vi "IV_RLJ_2015640305_P5.vi"(7 "OPERACIONES":T2(ring), 8 "Error In":errorcluster, 10 "OPERADORES":T1 {"y 2" scale=0.0..4.0; "Meter" scale=-360.0..360.0 scale format="%#_3g"; "y" scale=-150.0..150.0; "x" scale=-150.0..150.0}, 11 "IMAGEN 1":path) -> (0 "Error Out":errorcluster, 1 "HISTOGRAMA":dbl[][](graph), 2 "IMAGEN MODIFICADA":picture, 3 "IMAGEN ORIGINAL":picture)   [LabVIEW 2016]
doc: "subVI para la operacion sobre imagenes jpg, jpeg, o png que muestra el histograma RGB de la imagen modificada."
uses:
  <vilib>/picture/picture.llb/Draw True-Color Pixmap.vi
  <vilib>/imath/engines/lvmath2/RunTimeEngine/Managers/WorkSpace/UID Generator.vi
  <vilib>/imath/engines/lvmath2/RunTimeEngine/BuiltInFunctions/size/NIMS_[I32,I32]=size(GM).vi
  <instcachedir>/0/NIMS_[I32,I32]=size(GM)_B0A6EC1255BB4C8AB801FE6F734128D9.lvgen/NIMS_[I32,I32]=size(GM)_B0A6EC1255BB4C8AB801FE6F734128D9_005.vi
  <vilib>/imath/engines/lvmath2/RunTimeSupport/NIMS_Complex To Real.vi
  <instcachedir>/0/NIMS_Complex To Real_A9DD49CC305F495FA24B9F5762C73A31.lvgen/NIMS_Complex To Real_A9DD49CC305F495FA24B9F5762C73A31_001.vi
  <vilib>/imath/engines/lvmath2/RunTimeEngine/BuiltInFunctions/zeros/NIMS_M=zeros(I32,I32).vi
  <vilib>/imath/engines/lvmath2/RunTimeEngine/ErrorHandling/NIMS_Create Error From Enums.vi
  <vilib>/imath/engines/lvmath2/RunTimeEngine/RangeToken/NIMS_Range.vi
  <instcachedir>/0/NIMS_Range_A7C094595B484CA7AF10685B02D808ED.lvgen/NIMS_Range_A7C094595B484CA7AF10685B02D808ED_000.vi
  <vilib>/imath/engines/lvmath2/RunTimeSupport/NIMS_Error if Not Equal.vi
  <instcachedir>/0/NIMS_Error if Not Equal_43252A79AD05436189442EC0C5E5AB8A.lvgen/NIMS_Error if Not Equal_43252A79AD05436189442EC0C5E5AB8A_001.vi
  <vilib>/imath/engines/lvmath2/RunTimeEngine/IndexReplace/NIMS M(V,V)=M.vi
  <instcachedir>/0/NIMS M(V,V)=M_7C673E496ABD4677A4D7F51E7F4F45D1.lvgen/NIMS M(V,V)=M_7C673E496ABD4677A4D7F51E7F4F45D1_004.vi
  <vilib>/imath/engines/lvmath2/RunTimeEngine/BuiltInFunctions/size/NIMS_I32=size(GM,I32).vi
  <instcachedir>/0/NIMS_I32=size(GM,I32)_122058B1B3294FAEA5DC209B92B394E4.lvgen/NIMS_I32=size(GM,I32)_122058B1B3294FAEA5DC209B92B394E4_005.vi
  <vilib>/imathl/engines/lvmath/Functions/Error Handling/Create Error.vi
  <vilib>/imath/engines/lvmath2/RunTimeEngine/BuiltInFunctions/size/NIMS_I32Row=size(GM).vi
  <instcachedir>/0/NIMS_I32Row=size(GM)_10ACDCB9F1F84A7E9F42C91D87611FB5.lvgen/NIMS_I32Row=size(GM)_10ACDCB9F1F84A7E9F42C91D87611FB5_006.vi
  <vilib>/imath/engines/lvmath2/RunTimeEngine/BuiltInFunctions/zeros/NIMS_M=zeros(I32V).vi
  <vilib>/imath/engines/lvmath2/RunTimeEngine/RangeToken/NIMS_Range_R2 - Integer.vi
  <instcachedir>/0/NIMS_Range_R2 - Integer_89B873E74E6E489885E44F751DD9C6BF.lvgen/NIMS_Range_R2 - Integer_89B873E74E6E489885E44F751DD9C6BF_000.vi
  <vilib>/imath/engines/lvmath2/RunTimeEngine/CommandStatement/MC_CommandStatement_break.vi
  <vilib>/imath/engines/lvmath2/RunTimeEngine/BuiltInFunctions/round/NIMS_round(DBL-S).vi
  <instcachedir>/0/NIMS_Error if Not Equal_43252A79AD05436189442EC0C5E5AB8A.lvgen/NIMS_Error if Not Equal_43252A79AD05436189442EC0C5E5AB8A_000.vi
  <vilib>/imath/engines/lvmath2/RunTimeEngine/IndexRead/NIMS M(S,S).vi
  <instcachedir>/0/NIMS M(S,S)_AC51E74150A542F7991B9634C66F3096.lvgen/NIMS M(S,S)_AC51E74150A542F7991B9634C66F3096_002.vi
  <vilib>/imath/engines/lvmath2/RunTimeEngine/IndexReplace/NIMS M(S,S)=S.vi
  <instcachedir>/0/NIMS M(S,S)=S_98E40400474E4398B113AE20298B4F82.lvgen/NIMS M(S,S)=S_98E40400474E4398B113AE20298B4F82_003.vi
  <vilib>/imath/engines/lvmath2/RunTimeEngine/RunTimeType/NIMS_RunTimeType_From StrictType (excl LVString).vi
  <instcachedir>/0/NIMS_RunTimeType_From StrictType (excl LVString)_BBF44FB49F834B71AF7A14CCEDF8BECD.lvgen/NIMS_RunTimeType_From StrictType (excl LVString)_BBF44FB49F834B71AF7A14CCEDF8BECD_000.vi
  <vilib>/imath/engines/lvmath2/RunTimeEngine/LocalVariableDefStatement/MC_LocalVariableDefStatement_Display.vi
  <vilib>/imath/engines/lvmath2/RunTimeEngine/IndexRead/NIMS M(V,V).vi
  <instcachedir>/0/NIMS M(V,V)_DD7FAD36288F49D588C120E7830B6EC1.lvgen/NIMS M(V,V)_DD7FAD36288F49D588C120E7830B6EC1_005.vi
  <vilib>/imath/engines/lvmath2/RunTimeEngine/Managers/SymbolTable/Clear UID.vi
  <vilib>/imath/engines/lvmath2/RunTimeEngine/NodeEndStatement/NIMS_NodeEndStatement_Output.vi
  <instcachedir>/0/NIMS_NodeEndStatement_Output_53EC0D466D134D7ABD903AC30B43404B.lvgen/NIMS_NodeEndStatement_Output_53EC0D466D134D7ABD903AC30B43404B_010.vi
  <vilib>/imath/engines/lvmath2/RunTimeEngine/ErrorHandling/NIMS_Finalize Error.vi
  <vilib>/Analysis/Matrix/Numeric/Conversions/Array To Matrix - RA2.vi
  <vilib>/Analysis/Matrix/Numeric/Conversions/Matrix To Array - RM.vi
  <vilib>/imath/engines/lvmath2/RunTimeEngine/BuiltInFunctions/rotate90/NIMS_rotate90.vi
  <instcachedir>/0/NIMS_rotate90_7DC1660D109944E092D2EB6E3185A1B6.lvgen/NIMS_rotate90_7DC1660D109944E092D2EB6E3185A1B6_004.vi
  <vilib>/imath/engines/lvmath2/RunTimeEngine/IndexRead/NIMS M(R2,S).vi
  <instcachedir>/0/NIMS M(R2,S)_56813DCFDD5A484292D2195AF15D2BF5.lvgen/NIMS M(R2,S)_56813DCFDD5A484292D2195AF15D2BF5_000.vi
  <vilib>/imath/engines/lvmath2/RunTimeEngine/IndexReplace/NIMS M(R2,S)=V.vi
  <instcachedir>/0/NIMS M(R2,S)=V_4CAA475A15784754AE70E3CCB958AE2E.lvgen/NIMS M(R2,S)=V_4CAA475A15784754AE70E3CCB958AE2E_000.vi
  <instcachedir>/0/NIMS_NodeEndStatement_Output_53EC0D466D134D7ABD903AC30B43404B.lvgen/NIMS_NodeEndStatement_Output_53EC0D466D134D7ABD903AC30B43404B_002.vi
  <vilib>/Analysis/Matrix/NI_Matrix.lvlib
  <vilib>/imath/engines/lvmath2/RunTimeEngine/Managers/SymbolTable/NIMS_WorkSpace.lvlib
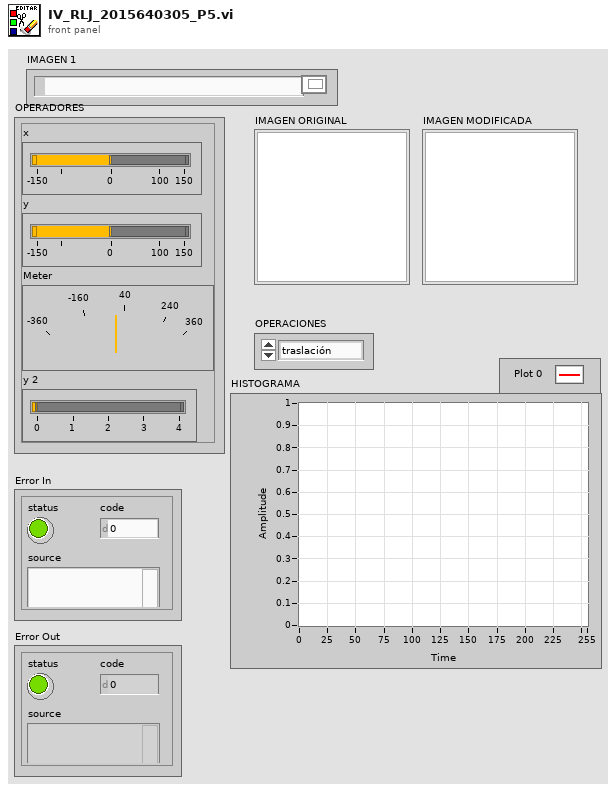
[diagram p1: front panel]
types:
  T1 = cluster{"x":dbl, "y":dbl, "Meter":dbl, "y 2":i64}
  T2 = enum16{"traslación", "Rotación", "Zoom", "GIROH", "GIROV", "Extracción", "Sustitución", "UNION"}
  T3 = typedef "imagedata.ctl" = cluster{"image type":i32, "image depth":i32, "image":u8[], "mask":u8[], "colors":u32[], "Rectangle":cluster{"left":i16, "top":i16, "right":i16, "bottom":i16}}
  T4 = typedef "NI_Matrix.lvlib/RealMatrix.ctl" = dbl[][]
  T5 = cluster{"left":i16, "top":i16, "right":i16, "bottom":i16}
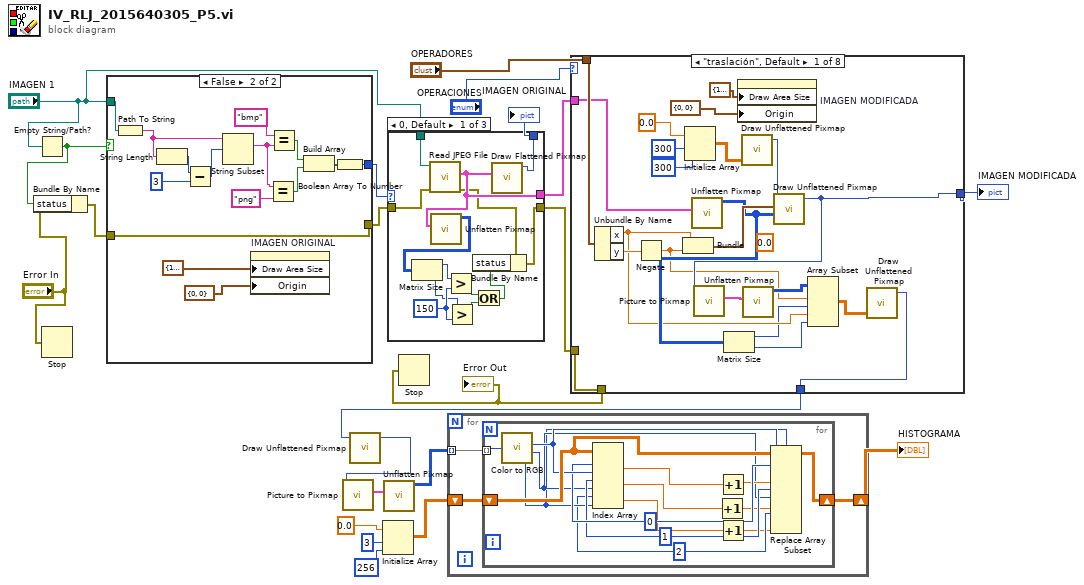
[diagram p0: block diagram]
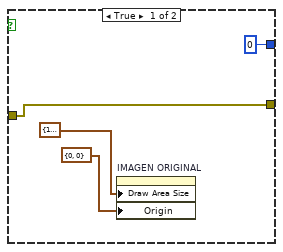
[diagram p2: hidden frame]
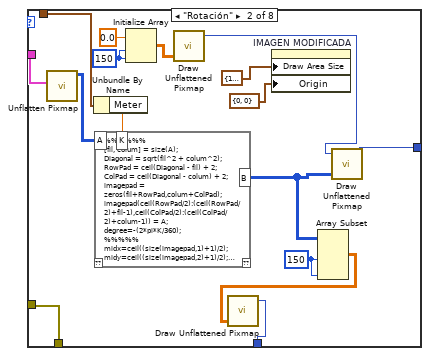
[diagram p3: hidden frame]
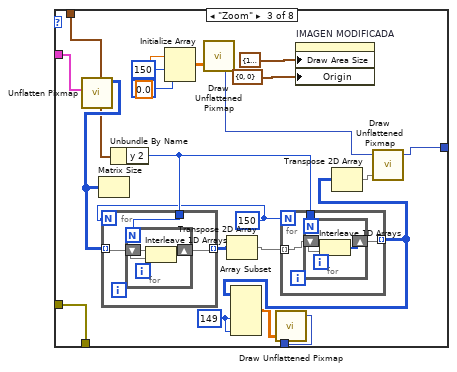
[diagram p4: hidden frame]
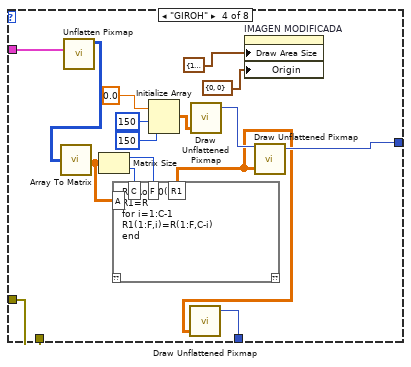
[diagram p5: hidden frame]
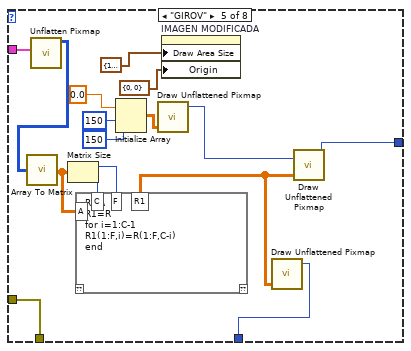
[diagram p6: hidden frame]
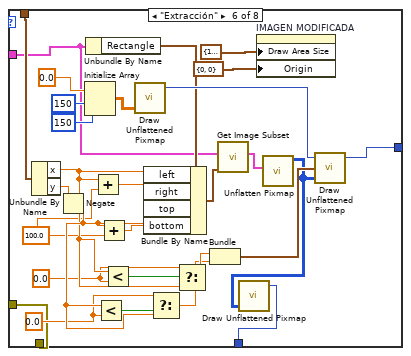
[diagram p7: hidden frame]
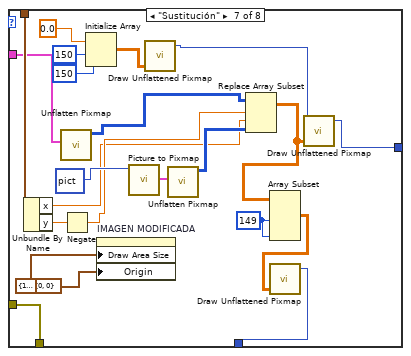
[diagram p8: hidden frame]
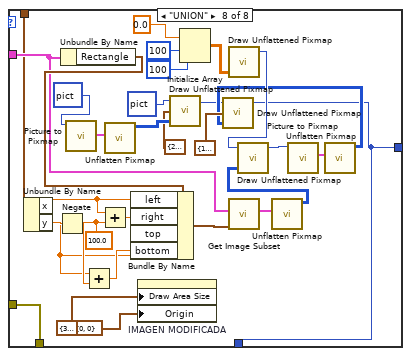
[diagram p9: hidden frame]
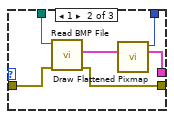
[diagram p10: hidden frame]
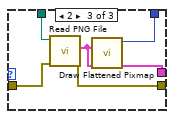
[diagram p11: hidden frame]
diagram:
  n1 = Empty String/Path?(string/path="IMAGEN 1") -> (empty?=w3:bool)
  n2 = Bundle By Name(cluster="Error In", "status"=w3) -> (w2:errorcluster)
  n3 = Stop(stop? (T)="Error In") -> ()
  n4 = case shown="False" w3 {
    tunnel: [u32 0 w36] -> w22
    tunnel: [w23 w27] -> w21
    tunnel: "IMAGEN 1" -> [_ w30]
    tunnel: w2 -> [w23 w27]
    frame True {
      n5 = property on="IMAGEN ORIGINAL" class="Pict"("Draw Area Size"=cluster{"Width":u32, "Height":u32} {"Width"=150, "Height"=150} ("Caption.Size"), "Origin"=cluster{"Horizontal":i16, "Vertical":i16} {"Horizontal"=0, "Vertical"=0}) -> ()  [unwired: 2 in, 2 out]
    }
    frame False {
      n6 = Path To String(path=w30) -> (string=w31:string)
      n7 = String Length(string=w31) -> (length=w41:i32)
      n8 = Subtract(x=w41, y=3) -> (x-y=w39:i32)
      n9 = String Subset(string=w31, offset (0)=w39) -> (substring=w32:string)  [unwired: 1 in]
      n10 = property on="IMAGEN ORIGINAL" class="Pict"("Draw Area Size"=cluster{"Width":u32, "Height":u32} {"Width"=150, "Height"=150} ("Caption.Size"), "Origin"=cluster{"Horizontal":i16, "Vertical":i16} {"Horizontal"=0, "Vertical"=0}) -> ()  [unwired: 2 in, 2 out]
      n11 = Equal?(x=w32, y="png" ("x")) -> (x = y?=w34:bool)
      n12 = Equal?(x="bmp", y=w32) -> (x = y?=w33:bool)
      n13 = Build Array(w33, w34) -> (w35:bool[])
      n14 = Boolean Array To Number(Boolean array=w35) -> (number=w36:u32)
    }
  }
  n15 = Initialize Array(0.0 ("element"), 3 ("dimension size"), 256 ("dimension size")) -> (w5:dbl[][])
  n16 = case shown="0, Default" w22 {
    tunnel: "IMAGEN 1" -> [w54 w59 w64]
    tunnel: [w51 w58 w63] -> w20
    tunnel: w21 -> [w53 w57 w62]
    tunnel: [w42 w56 w61] -> w15
    tunnel: [w52 w55 w60] -> w19
    frame 0, Default {
      w47 = 150 ("y")
      n17 = call <vilib>:"Read JPEG File.vi"("error in (no error)"=w53, "path to JPEG file"=w54) -> ("error out"=w43:errorcluster, "image data"=w51:T3)  [unwired: 7 in, 1 out]
      n18 = call <vilib>:"Unflatten Pixmap.vi"("image data"=w51) -> ("24-bit pixmap"=w50:u32[][])  [unwired: 4 in, 6 out]
      n19 = Matrix Size(0:w50) -> (1:w46:i32, 2:w45:i32)
      n20 = Greater?(x=w46, y=w47) -> (0:w48:bool)
      n21 = Greater?(x=w45, y=w47) -> (0:w49:bool)
      n22 = Or(x=w48, y=w49) -> (x .or. y?=w44:bool)
      n23 = Bundle By Name(cluster=w43, "status"=w44) -> (w42:errorcluster)
      n24 = call <vilib>:"Draw Flattened Pixmap.vi"("image data"=w51) -> ("new picture"=w52:picture)  [unwired: 8 in]
    }
    frame 1 {
      n25 = call <vilib>:"Read BMP File.vi"("error in (no error)"=w57, "path to BMP file"=w59) -> ("error out"=w56:errorcluster, "image data"=w58:T3)  [unwired: 7 in, 1 out]
      n26 = call <vilib>:"Draw Flattened Pixmap.vi"("image data"=w58) -> ("new picture"=w55:picture)  [unwired: 8 in]
    }
    frame 2 {
      n27 = call <vilib>:"Read PNG File.vi"("error in (no error)"=w62, "path to PNG file"=w64) -> ("error out"=w61:errorcluster, "image data"=w63:T3)  [unwired: 7 in, 1 out]
      n28 = call <vilib>:"Draw Flattened Pixmap.vi"("image data"=w63) -> ("new picture"=w60:picture)  [unwired: 8 in]
    }
  }
  "IMAGEN ORIGINAL" <- w19
  n29 = case shown="\"traslación\", Default" "OPERACIONES" {
    tunnel: [w75 w102 w699 w729 w894 w1032 w1059 w1081] -> w18
    tunnel: w20 -> [w81 w100 w700 w728 w888 w1033 w1071 w1109]
    tunnel: "OPERADORES" -> [w82 w101 w701 _ _ w1034 w1080 w1105]
    tunnel: w15 -> [w80 w97 w713 w739 w881 w1035 w1070 w1082]
    tunnel: [w80 w97 w713 w739 w881 w1035 w1070 w1082] -> w14
    tunnel: [w71 w91 w698 w726 w879 w1030 w1060 w1081] -> w13
    frame "traslación", Default {
      (unwired) 0.0 ("t")
      n30 = Unbundle By Name(w82) -> ("x"=w67:dbl, "y"=w77:dbl)
      n31 = Negate(x=w77) -> (-x=w66:dbl)
      n32 = Bundle("x"=w67, w66) -> (w70:cluster{"x":dbl, dbl})  [unwired: 1 in]
      n33 = Initialize Array(0.0 ("element"), 300 ("dimension size"), 300 ("dimension size")) -> (w83:dbl[][])
      n34 = call <vilib>:"Unflatten Pixmap.vi"("image data"=w81) -> ("24-bit pixmap"=w69:u32[][])  [unwired: 4 in, 6 out]
      n35 = Matrix Size(0:w69) -> (1:w65:i32, 2:w68:i32)
      n36 = property on="IMAGEN MODIFICADA" class="Pict"("Draw Area Size"=cluster{"Width":u32, "Height":u32} {"Width"=150, "Height"=150} ("Caption.Size"), "Origin"=cluster{"Horizontal":i16, "Vertical":i16} {"Horizontal"=0, "Vertical"=0}) -> ()  [unwired: 2 in, 2 out]
      n37 = call-poly <vilib>:"Draw Unflattened Pixmap.vi"("data (RGB format)"=w83) -> ("new picture"=w76:picture)  [unwired: 8 in]
      n38 = call-poly <vilib>:"Draw Unflattened Pixmap.vi"("picture"=w76, "top left point(0, 0)"=w70, "data (RGB format)"=w69) -> ("new picture"=w75:picture)  [unwired: 6 in]
      n39 = call <vilib>:"Picture to Pixmap.vi"("picture"=w75) -> ("image data"=w74:T3)  [unwired: 9 in, 1 out]
      n40 = call <vilib>:"Unflatten Pixmap.vi"("image data"=w74) -> ("24-bit pixmap"=w73:u32[][])  [unwired: 4 in, 6 out]
      n41 = Array Subset(array=w73, index (row)=w66, length (row)=w65, index (col)=w67, length (col)=w68) -> (w72:dbl[][])
      n42 = call-poly <vilib>:"Draw Unflattened Pixmap.vi"("data (RGB format)"=w72) -> ("new picture"=w71:picture)  [unwired: 8 in]
    }
    frame "Rotación" {
      w90 = 150 ("row N")
      w96 = 150 ("dimension size")
      n43 = call <vilib>:"Unflatten Pixmap.vi"("image data"=w100) -> ("24-bit pixmap"=w92:u32[][])  [unwired: 4 in, 6 out]
      n44 = Unbundle By Name(w101) -> ("Meter"=w93:dbl)
      n45 = mathscript code="%%%%%%\n[fil, colum] = size(A); \nDiagonal = sqrt(fil^2 + colum^2); \nRowPad = ceil(Diagonal - fil) + 2;\nColPad = ceil(Diagonal - colum) + 2;\nimagepad = zeros(fil+RowPad,colum+ColPad);\nimagepad(ceil(RowPad/2):(ceil(RowPad/2)+fil-1),ceil(ColPad/2):(ceil(ColPad/2)+colum-1)) = A;\ndegree=-(2*pi*K/360);\n%%%%%\nmidx=ceil((size(imagepad,1)+1)/2);\nmidy=ceil((size(imagepad,2)+1)/2);\nB=zeros(size(imagepad));\n%%%%%%\nfor i=1:size(imagepad,1)\n    for j=1:size(imagepad,2)\n         x=(i-midx)*cos(degree)-(j-midy)*sin(degree);\n         y=(i-midx)*sin(degree)+(j-midy)*cos(degree);\n         x=round(x)+midx;\n         y=round(y)+midy;\n         if (x>=1 && y>=1)\n             B(x,y)=imagepad(i,j);        \n         end\n    end\nend\n[m1,n1]=size(imagepad)\n[m,n]=size(B)\nPY=ceil((m1-fil)/2)\nPX=ceil((n1-colum)/2)\nB=B(PY:m,PX:n)"("K"=w93, "A"=w92) -> ("B"=w89:u32[][])  [unwired: 1 in, 1 out]
      n46 = Initialize Array(0.0 ("element"), w96, w96) -> (w94:dbl[][])
      n47 = call-poly <vilib>:"Draw Unflattened Pixmap.vi"("data (RGB format)"=w94) -> ("new picture"=w87:picture)  [unwired: 8 in]
      n48 = property on="IMAGEN MODIFICADA" class="Pict"("Draw Area Size"=cluster{"Width":u32, "Height":u32} {"Width"=150, "Height"=150} ("Caption.Size"), "Origin"=cluster{"Horizontal":i16, "Vertical":i16} {"Horizontal"=0, "Vertical"=0}) -> ()  [unwired: 2 in, 2 out]
      n49 = Array Subset(array=w89, length (row)=w90, length (col)=w90) -> (w88:dbl[][])  [unwired: 2 in]
      n50 = call-poly <vilib>:"Draw Unflattened Pixmap.vi"("data (RGB format)"=w88) -> ("new picture"=w91:picture)  [unwired: 8 in]
      n51 = call-poly <vilib>:"Draw Unflattened Pixmap.vi"("picture"=w87, "data (RGB format)"=w89) -> ("new picture"=w102:picture)  [unwired: 7 in]
    }
    frame "Zoom" {
      w695 = 149 ("row N")
      w703 = 150
      n52 = call <vilib>:"Unflatten Pixmap.vi"("image data"=w700) -> ("24-bit pixmap"=w702:u32[][])  [unwired: 4 in, 6 out]
      n53 = Matrix Size(0:w702) -> ()  [unwired: 2 out]
      n54 = Unbundle By Name(w701) -> ("y 2"=w705:i64)
      n55 = for {
        N: w703 -> [_]
        tunnel: w702 -> [w723] mode=indexing
        tunnel: w705 -> [w722]
        tunnel: [w721] -> w707 mode=indexing
        n56 = for {
          N: w722 -> [_]
          shift-right: [w724] -> w721
          shift-left: w723 -> [w725]
          n57 = Interleave 1D Arrays(w725, w725) -> (w724:u32[])
        }
      }
      n58 = Initialize Array(0.0 ("element"), 150 ("dimension size"), 150 ("dimension size")) -> (w709:dbl[][])
      n59 = call-poly <vilib>:"Draw Unflattened Pixmap.vi"("data (RGB format)"=w709) -> ("new picture"=w708:picture)  [unwired: 8 in]
      n60 = Transpose 2D Array(2D array=w707) -> (transposed array=w706:u32[][])
      n61 = for {
        N: w703 -> [_]
        tunnel: w705 -> [w718]
        tunnel: [w717] -> w697 mode=indexing
        tunnel: w706 -> [w716] mode=indexing
        n62 = for {
          N: w718 -> [_]
          shift-right: [w719] -> w717
          shift-left: w716 -> [w720]
          n63 = Interleave 1D Arrays(w720, w720) -> (w719:u32[])
        }
      }
      n64 = Array Subset(array=w697, length (row)=w695, length (col)=w695) -> (w696:dbl[][])  [unwired: 2 in]
      n65 = call-poly <vilib>:"Draw Unflattened Pixmap.vi"("data (RGB format)"=w696) -> ("new picture"=w698:picture)  [unwired: 8 in]
      n66 = property on="IMAGEN MODIFICADA" class="Pict"("Draw Area Size"=cluster{"Width":u32, "Height":u32} {"Width"=150, "Height"=150} ("Caption.Size"), "Origin"=cluster{"Horizontal":i16, "Vertical":i16} {"Horizontal"=0, "Vertical"=0}) -> ()  [unwired: 2 in, 2 out]
      n67 = Transpose 2D Array(2D array=w697) -> (transposed array=w704:u32[][])
      n68 = call-poly <vilib>:"Draw Unflattened Pixmap.vi"("picture"=w708, "data (RGB format)"=w704) -> ("new picture"=w699:picture)  [unwired: 7 in]
    }
    frame "GIROH" {
      n69 = call <vilib>:"Unflatten Pixmap.vi"("image data"=w728) -> ("24-bit pixmap"=w733:u32[][])  [unwired: 4 in, 6 out]
      n70 = call-poly <vilib>:"Array To Matrix.vi"("Real 2D Array"=w733) -> ("Real Matrix"=w730:T4)
      n71 = Matrix Size(0:w730) -> (1:w731:i32, 2:w738:i32)
      n72 = mathscript code="R=Rot90(A,2)\nR1=R\nfor i=1:C-1\nR1(1:F,i)=R(1:F,C-i)\nend"("A"=w730, "C"=w738, "F"=w731) -> ("R1"=w727:dbl[][])  [unwired: 1 in, 1 out]
      n73 = Initialize Array(0.0 ("element"), 150 ("dimension size"), 150 ("dimension size")) -> (w734:dbl[][])
      n74 = call-poly <vilib>:"Draw Unflattened Pixmap.vi"("data (RGB format)"=w727) -> ("new picture"=w726:picture)  [unwired: 8 in]
      n75 = call-poly <vilib>:"Draw Unflattened Pixmap.vi"("data (RGB format)"=w734) -> ("new picture"=w732:picture)  [unwired: 8 in]
      n76 = property on="IMAGEN MODIFICADA" class="Pict"("Draw Area Size"=cluster{"Width":u32, "Height":u32} {"Width"=150, "Height"=150} ("Caption.Size"), "Origin"=cluster{"Horizontal":i16, "Vertical":i16} {"Horizontal"=0, "Vertical"=0}) -> ()  [unwired: 2 in, 2 out]
      n77 = call-poly <vilib>:"Draw Unflattened Pixmap.vi"("picture"=w732, "data (RGB format)"=w727) -> ("new picture"=w729:picture)  [unwired: 7 in]
    }
    frame "GIROV" {
      n78 = call <vilib>:"Unflatten Pixmap.vi"("image data"=w888) -> ("24-bit pixmap"=w887:u32[][])  [unwired: 4 in, 6 out]
      n79 = call-poly <vilib>:"Array To Matrix.vi"("Real 2D Array"=w887) -> ("Real Matrix"=w884:T4)
      n80 = Matrix Size(0:w884) -> (1:w885:i32, 2:w893:i32)
      n81 = mathscript code="R=A\nR1=R\nfor i=1:C-1\nR1(1:F,i)=R(1:F,C-i)\nend"("A"=w884, "C"=w893, "F"=w885) -> ("R1"=w880:dbl[][])  [unwired: 1 in, 1 out]
      n82 = Initialize Array(0.0 ("element"), 150 ("dimension size"), 150 ("dimension size")) -> (w889:dbl[][])
      n83 = call-poly <vilib>:"Draw Unflattened Pixmap.vi"("data (RGB format)"=w889) -> ("new picture"=w886:picture)  [unwired: 8 in]
      n84 = property on="IMAGEN MODIFICADA" class="Pict"("Draw Area Size"=cluster{"Width":u32, "Height":u32} {"Width"=150, "Height"=150} ("Caption.Size"), "Origin"=cluster{"Horizontal":i16, "Vertical":i16} {"Horizontal"=0, "Vertical"=0}) -> ()  [unwired: 2 in, 2 out]
      n85 = call-poly <vilib>:"Draw Unflattened Pixmap.vi"("data (RGB format)"=w880) -> ("new picture"=w879:picture)  [unwired: 8 in]
      n86 = call-poly <vilib>:"Draw Unflattened Pixmap.vi"("picture"=w886, "data (RGB format)"=w880) -> ("new picture"=w894:picture)  [unwired: 7 in]
    }
    frame "Extracción" {
      w1053 = 0.0 ("y")
      w1052 = 0.0 ("y")
      w1048 = 100.0 ("y")
      n87 = Unbundle By Name(w1034) -> ("x"=w1057:dbl, "y"=w1050:dbl)
      n88 = Negate(x=w1050) -> (-x=w1058:dbl)
      n89 = Initialize Array(0.0 ("element"), 150 ("dimension size"), 150 ("dimension size")) -> (w1044:dbl[][])
      n90 = Unbundle By Name(w1033) -> ("Rectangle"=w1036:T5)
      n91 = Add(x=w1057, y=w1048) -> (x+y=w1039:dbl)
      n92 = Less?(x=w1058, y=w1052) -> (x < y?=w1049:bool)
      n93 = Add(x=w1058, y=w1048) -> (x+y=w1038:dbl)
      n94 = Less?(x=w1057, y=w1053) -> (x < y?=w1054:bool)
      n95 = call-poly <vilib>:"Draw Unflattened Pixmap.vi"("data (RGB format)"=w1044) -> ("new picture"=w1045:picture)  [unwired: 8 in]
      n96 = Bundle By Name(cluster=w1036, "left"=w1057, "right"=w1039, "top"=w1058, "bottom"=w1038) -> (w1037:T5)
      n97 = Select(t=w1052, s=w1049, f=w1058) -> (s? t:f=w1051:dbl)
      n98 = Select(t=w1053, s=w1054, f=w1057) -> (s? t:f=w1055:dbl)
      n99 = Bundle("x"=w1055, "y"=w1051) -> (w1056:cluster{"x":dbl, "y":dbl})  [unwired: 1 in]
      n100 = call <vilib>:"Get Image Subset.vi"("subset rect"=w1037, "image data"=w1033) -> ("image subset"=w1040:T3)  [unwired: 4 in, 1 out]
      n101 = property on="IMAGEN MODIFICADA" class="Pict"("Draw Area Size"=cluster{"Width":u32, "Height":u32} {"Width"=150, "Height"=150} ("Caption.Size"), "Origin"=cluster{"Horizontal":i16, "Vertical":i16} {"Horizontal"=0, "Vertical"=0}) -> ()  [unwired: 2 in, 2 out]
      n102 = call <vilib>:"Unflatten Pixmap.vi"("image data"=w1040) -> ("24-bit pixmap"=w1031:u32[][])  [unwired: 4 in, 6 out]
      n103 = call-poly <vilib>:"Draw Unflattened Pixmap.vi"("data (RGB format)"=w1031) -> ("new picture"=w1030:picture)  [unwired: 8 in]
      n104 = call-poly <vilib>:"Draw Unflattened Pixmap.vi"("picture"=w1045, "top left point(0, 0)"=w1056, "data (RGB format)"=w1031) -> ("new picture"=w1032:picture)  [unwired: 6 in]
    }
    frame "Sustitución" {
      w1062 = 149 ("row N")
      n105 = Unbundle By Name(w1080) -> ("x"=w1064:dbl, "y"=w1076:dbl)
      n106 = call <vilib>:"Unflatten Pixmap.vi"("image data"=w1071) -> ("24-bit pixmap"=w1068:u32[][])  [unwired: 4 in, 6 out]
      n107 = Negate(x=w1076) -> (-x=w1065:dbl)
      n108 = Initialize Array(0.0 ("element"), 150 ("dimension size"), 150 ("dimension size")) -> (w1072:dbl[][])
      n109 = property on="IMAGEN MODIFICADA" class="Pict"("Draw Area Size"=cluster{"Width":u32, "Height":u32} {"Width"=150, "Height"=150} ("Caption.Size"), "Origin"=cluster{"Horizontal":i16, "Vertical":i16} {"Horizontal"=0, "Vertical"=0}) -> ()  [unwired: 2 in, 2 out]
      n110 = call <vilib>:"Picture to Pixmap.vi"("picture"=picture bytes[30030] ("IMAGEN ORIGINAL 2")) -> ("image data"=w1075:T3)  [unwired: 9 in, 1 out]
      n111 = call-poly <vilib>:"Draw Unflattened Pixmap.vi"("data (RGB format)"=w1072) -> ("new picture"=w1066:picture)  [unwired: 8 in]
      n112 = call <vilib>:"Unflatten Pixmap.vi"("image data"=w1075) -> ("24-bit pixmap"=w1067:u32[][])  [unwired: 4 in, 6 out]
      n113 = Replace Array Subset(array=w1068, new element=w1067, index (row)=w1065, index (col)=w1064) -> (w1063:T4)
      n114 = Array Subset(array=w1063, length (row)=w1062, length (col)=w1062) -> (w1061:T4)  [unwired: 2 in]
      n115 = call-poly <vilib>:"Draw Unflattened Pixmap.vi"("data (RGB format)"=w1061) -> ("new picture"=w1060:picture)  [unwired: 8 in]
      n116 = call-poly <vilib>:"Draw Unflattened Pixmap.vi"("picture"=w1066, "data (RGB format)"=w1063) -> ("new picture"=w1059:picture)  [unwired: 7 in]
    }
    frame "UNION" {
      w1100 = 100.0 ("y")
      n117 = Unbundle By Name(w1105) -> ("x"=w1091:dbl, "y"=w1099:dbl)
      n118 = Negate(x=w1099) -> (-x=w1092:dbl)
      n119 = Unbundle By Name(w1109) -> ("Rectangle"=w1111:T5)
      n120 = call <vilib>:"Picture to Pixmap.vi"("picture"=picture bytes[30030] ("new picture 3")) -> ("image data"=w1098:T3)  [unwired: 9 in, 1 out]
      n121 = Add(x=w1092, y=w1100) -> (x+y=w1108:dbl)
      n122 = Add(x=w1091, y=w1100) -> (x+y=w1107:dbl)
      n123 = call <vilib>:"Unflatten Pixmap.vi"("image data"=w1098) -> ("24-bit pixmap"=w1097:u32[][])  [unwired: 4 in, 6 out]
      n124 = Bundle By Name(cluster=w1111, "left"=w1091, "right"=w1107, "top"=w1092, "bottom"=w1108) -> (w1110:T5)
      n125 = property on="IMAGEN MODIFICADA" class="Pict"("Draw Area Size"=cluster{"Width":u32, "Height":u32} {"Width"=300, "Height"=100} ("Caption.Size"), "Origin"=cluster{"Horizontal":i16, "Vertical":i16} {"Horizontal"=0, "Vertical"=0}) -> ()  [unwired: 2 in, 2 out]
      n126 = call-poly <vilib>:"Draw Unflattened Pixmap.vi"("picture"=picture bytes[30030] ("new picture 3"), "top left point(0, 0)"=cluster{"x":i16, "y":i16} {"x"=200, "y"=0}, "data (RGB format)"=w1097) -> ("new picture"=w1083:picture)  [unwired: 6 in]
      n127 = Initialize Array(0.0 ("element"), 100 ("dimension size"), 100 ("dimension size")) -> (w1101:dbl[][])
      n128 = call-poly <vilib>:"Draw Unflattened Pixmap.vi"("data (RGB format)"=w1101) -> ("new picture"=w1086:picture)  [unwired: 8 in]
      n129 = call <vilib>:"Get Image Subset.vi"("subset rect"=w1110, "image data"=w1109) -> ("image subset"=w1106:T3)  [unwired: 4 in, 1 out]
      n130 = call <vilib>:"Unflatten Pixmap.vi"("image data"=w1106) -> ("24-bit pixmap"=w1087:u32[][])  [unwired: 4 in, 6 out]
      n131 = call-poly <vilib>:"Draw Unflattened Pixmap.vi"("picture"=w1086, "data (RGB format)"=w1087) -> ("new picture"=w1085:picture)  [unwired: 7 in]
      n132 = call <vilib>:"Picture to Pixmap.vi"("picture"=w1085) -> ("image data"=w1095:T3)  [unwired: 9 in, 1 out]
      n133 = call <vilib>:"Unflatten Pixmap.vi"("image data"=w1095) -> ("24-bit pixmap"=w1084:u32[][])  [unwired: 4 in, 6 out]
      n134 = call-poly <vilib>:"Draw Unflattened Pixmap.vi"("picture"=w1083, "top left point(0, 0)"=cluster{"x":i16, "y":i16} {"x"=100, "y"=0}, "data (RGB format)"=w1084) -> ("new picture"=w1081:picture)  [unwired: 6 in]
    }
  }
  "Error Out" <- w14
  "IMAGEN MODIFICADA" <- w18
  n135 = call-poly <vilib>:"Draw Unflattened Pixmap.vi"("picture"=w13) -> ("new picture"=w12:picture)  [unwired: 8 in]
  n136 = call <vilib>:"Picture to Pixmap.vi"("picture"=w12) -> ("image data"=w11:T3)  [unwired: 9 in, 1 out]
  n137 = call <vilib>:"Unflatten Pixmap.vi"("image data"=w11) -> ("24-bit pixmap"=w10:u32[][])  [unwired: 4 in, 6 out]
  n138 = Stop(stop? (T)=w14) -> ()
  n139 = for {
    tunnel: w10 -> [w1114] mode=indexing
    shift-right: [w1112] -> w6
    shift-left: w5 -> [w1113]
    n140 = for {
      tunnel: w1114 -> [w1129] mode=indexing
      shift-right: [w1128] -> w1112
      shift-left: w1113 -> [w1127]
      w1117 = 2
      w1121 = 1
      w1124 = 0 ("disabled index (row)")
      n141 = call <vilib>:"Color to RGB.vi"("Color"=w1129) -> ("R"=w1125:u8, "G"=w1119:u8, "B"=w1118:u8)  [unwired: 1 out]
      n142 = Index Array(array=w1127, index (row) #1=w1124, index (col) #1=w1125, index (row) #2=w1121, index (col) #2=w1119, index (row) #3=w1117, index (col) #3=w1118) -> (element #1=w1126:dbl, element #2=w1123:dbl, element #3=w1116:dbl)
      n143 = Increment(x=w1123) -> (x+1=w1120:dbl)
      n144 = Increment(x=w1126) -> (x+1=w1122:dbl)
      n145 = Increment(x=w1116) -> (x+1=w1115:dbl)
      n146 = Replace Array Subset(array=w1127, new element #1=w1122, index (row) #1=w1124, index (col) #1=w1125, new element #2=w1120, index (row) #2=w1121, index (col) #2=w1119, new element #3=w1115, index (row) #3=w1117, index (col) #3=w1118) -> (w1128:dbl[][])
    }
  }
  "HISTOGRAMA" <- w6
